vi "Open_Multi_VI_Instances.vi"() -> ()   [LabVIEW 2011]
uses:
  GlobalStop.vi
panel:
  out "error out":errorcluster
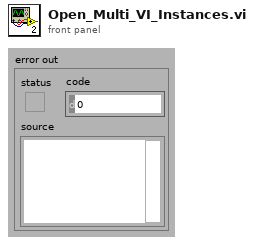
[diagram p1: front panel]
types:
  T1 = enum32{"Invalid", "Standard", "Closed", "Hidden", "Minimized", "Maximized"}
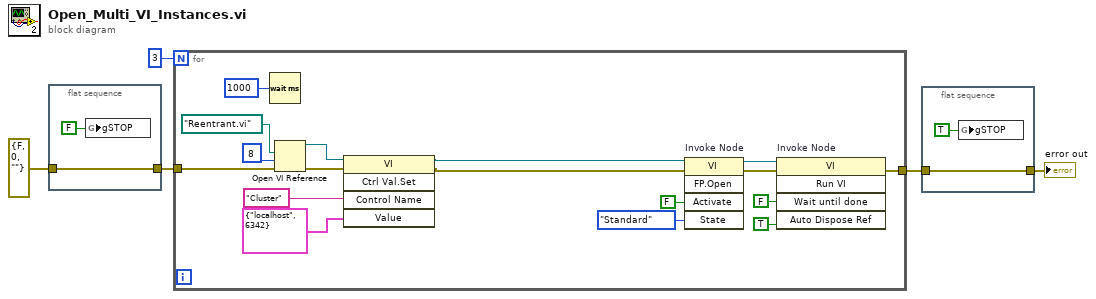
[diagram p0: block diagram]
diagram:
  n1 = flat-sequence {
    tunnel: errorcluster {"status"=FALSE, "code"=0, "source"=""} ("error constant") -> [w6]
    tunnel: [w6] -> w2
    frame #0 {
      n2 = global write "GlobalStop.vi" "gSTOP"(FALSE ("gSTOP")) -> ()
    }
  }
  n3 = for {
    N: 3 -> [_]
    tunnel: [w24] -> w4
    tunnel: w2 -> [w11]
    n4 = Wait (ms)(milliseconds to wait=u32 1000) -> ()  [unwired: 1 out]
    n5 = Open VI Reference(vi path=path "Reentrant.vi", options=8, error in (no error)=w11) -> (vi reference=w14:refnum<vi>, error out=w13:errorcluster)  [unwired: 3 out]
    n6 = invoke class="VI" method="Ctrl Val.Set"(reference=w14, error in=w13, "Control Name"="Cluster", "Value"=cluster{string, i32} {"localhost", 6342}) -> (reference out=w9:refnum<vi>, error out=w8:errorcluster)  [unwired: 1 in, 3 out]
    n7 = invoke on="Invoke Node" class="VI" method="FP.Open"(reference=w9, error in=w8, "Activate"=FALSE ("Activate?"), "State"=T1."Standard") -> (reference out=w21:refnum<vi>, error out=w20:errorcluster)  [unwired: 1 in, 3 out]
    n8 = invoke on="Invoke Node" class="VI" method="Run VI"(reference=w21, error in=w20, "Wait until done"=FALSE ("Wait Until Done"), "Auto Dispose Ref"=TRUE ("Auto Dispose Reference")) -> (error out=w24:errorcluster)  [unwired: 1 in, 4 out]
  }
  n9 = flat-sequence {
    tunnel: w4 -> [w25]
    tunnel: [w25] -> w3
    frame #0 {
      n10 = global write "GlobalStop.vi" "gSTOP"(TRUE ("gSTOP")) -> ()
    }
  }
  "error out" <- w3
